vi "Get Service Class Instances.vi"() -> (3 "service instances":refnum<class "ServiceBase.lvclass">[](array[class]))   [LabVIEW 2023, in "Generated_server.lvlib"]
uses:
  Generated_server.lvlib
  <vilib>/gRPC/LabVIEW gRPC Servicer/ServiceBase/ServiceBase.lvclass
  RPC Service/streamai/streamai.lvclass
  C:/Program Files (x86)/National Instruments/LabVIEW 2023/vi.lib/gRPC/LabVIEW gRPC Servicer/ServiceBase/ServiceBase.lvclass
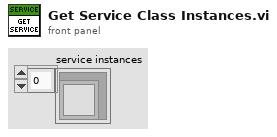
[diagram p1: front panel]
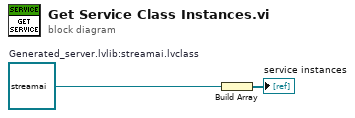
[diagram p0: block diagram]
diagram:
  w1 = refnum<class "streamai.lvclass"> refnum  # Generated_server.lvlib:streamai.lvclass
  n1 = Build Array(w1) -> (→"service instances":refnum<class "streamai.lvclass">[])
